vi "1 channel N  sample API( data reading).vi"() -> ()   [LabVIEW 2020]
uses:
  <vilib>/DAQmx/read.llb/DAQmx Read (Analog 1D DBL 1Chan NSamp).vi
  <vilib>/DAQmx/create/channels.llb/DAQmx Create Channel (AI-Temperature-Thermocouple).vi
  <vilib>/DAQmx/configure/timing.llb/DAQmx Timing (Sample Clock).vi
  <vilib>/DAQmx/miscellaneous.llb/DAQmx Fill In Error Info.vi
panel:
  in  "location":string
  in  "sensor name":string
  in  "sampling rate":string
  in  "Reasearch center name":string
  in  "Scientist name":string
  out "Waveform Graph":dbl[](graph)
  in  "number of samples per channel( user defined to read from the daq)":i32=-1
  out "Array":dbl[](array[numeric]) format="%0.2f"
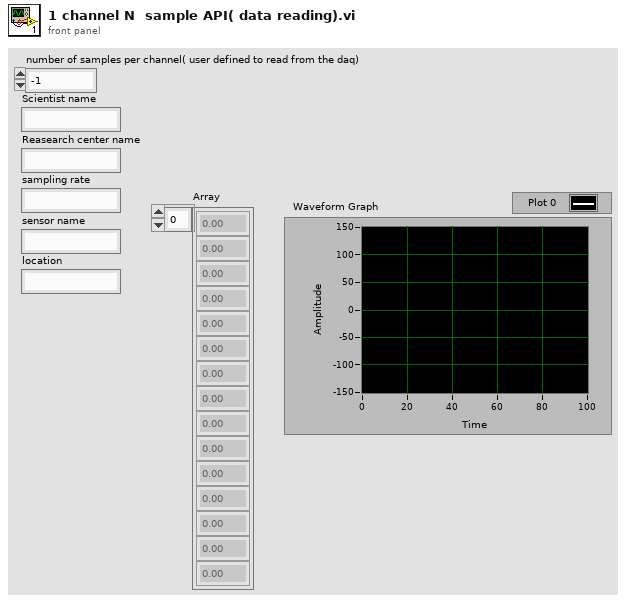
[diagram p1: front panel]
types:
  T1 = enum16{"open", "replace", "create", "open or create", "replace or create", "replace or create with confirmation"}
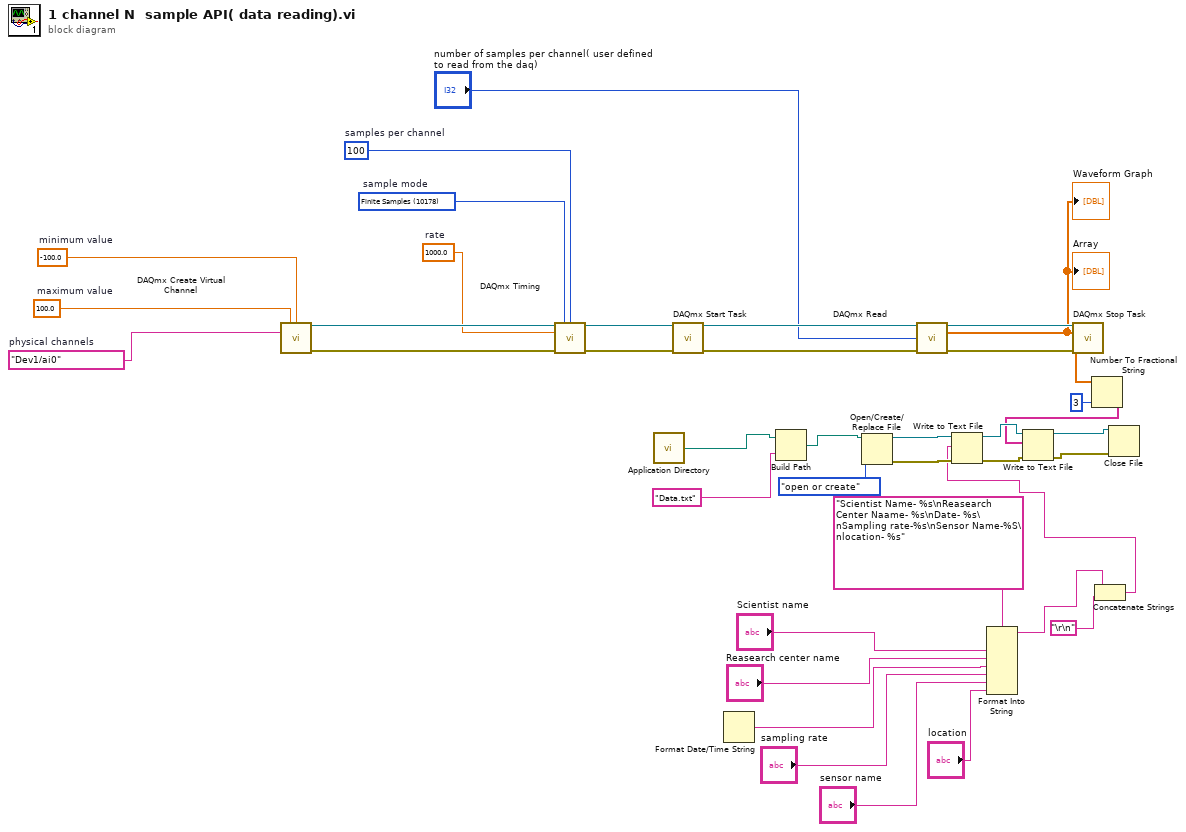
[diagram p0: block diagram]
diagram:
  w25 = 1000.0  # rate
  w28 = 10178 items=["Finite Samples"=10178, "Continuous Samples"=10123, "Hardware Timed Single Point"=12522]  # sample mode
  w29 = 100  # samples per channel
  w30 = 100.0  # maximum value
  w31 = -100.0  # minimum value
  w32 = tag "Dev1/ai0"  # physical channels
  n1 = call-poly <vilib>:"DAQmx Create Virtual Channel.vi"("maximum value"=w30, "minimum value"=w31, "physical channels"=w32) -> ("task out"=w27:refnum<k21>, "error out"=w36:errorcluster)  [unwired: 11 in]
  n2 = call-poly <vilib>:"DAQmx Timing.vi"("task/channels in"=w27, "sample mode"=w28, "samples per channel"=w29, "rate"=w25, "error in"=w36) -> ("task out"=w26:refnum<k21>, "error out"=w35:errorcluster)  [unwired: 9 in]
  n3 = call <vilib>:"Application Directory.vi"() -> ("Application Directory"=w23:path)
  n4 = call <vilib>:"DAQmx Start Task.vi"("task/channels in"=w26, "error in"=w35) -> ("task out"=w38:refnum<k21>, "error out"=w34:errorcluster)  [unwired: 12 in]
  n5 = Format Date/Time String() -> (date/time string=w4:string)  [unwired: 3 in]
  n6 = Build Path(base path=w23, name or relative path="Data.txt") -> (appended path=w21:path)
  n7 = Open/Create/Replace File(file path (use dialog)=w21, operation (0:open)=T1."open or create") -> (refnum out=w19:refnum<file>, error out=w18:errorcluster)  [unwired: 4 in, 1 out]
  n8 = call-poly <vilib>:"DAQmx Read.vi"("task/channels in"=w38, "number of samples per channel"="number of samples per channel( user defined to read from the daq)", "error in"=w34) -> ("task out"=w37:refnum<k21>, "data"=w13:dbl[], "error out"=w33:errorcluster)  [unwired: 10 in]
  "Array" <- w13
  "Waveform Graph" <- w13
  n9 = Format Into String(format string="Scientist Name- %s\nReasearch Center Naame- %s\nDate- %s\nSampling rate-%s\nSensor Name-%S\nlocation- %s", "Scientist name", "Reasearch center name", w4, "sampling rate", "sensor name", "location") -> (resulting string=w9:string)  [unwired: 2 in, 1 out]
  n10 = call <vilib>:"DAQmx Stop Task.vi"("task/channels in"=w37, "error in"=w33) -> ()  [unwired: 12 in, 2 out]
  n11 = Number To Fractional String(number=w13, precision (6)=i16 3) -> (F-format string=w12:string[])  [unwired: 2 in]
  n12 = Concatenate Strings(w9, "\r\n") -> (w8:string)
  n13 = Write to Text File(file (use dialog)=w19, text=w8, error in=w18) -> (refnum out=w17:refnum<file>, error out=w15:errorcluster)  [unwired: 1 in, 1 out]
  n14 = Write to Text File(file (use dialog)=w17, text=w12, error in=w15) -> (refnum out=w16:refnum<file>, error out=w14:errorcluster)  [unwired: 1 in, 1 out]
  n15 = Close File(refnum=w16, error in=w14) -> ()  [unwired: 2 out]
